vi "2023_day10_Task2.vi"() -> ()   [LabVIEW 2021]
uses:
  458e69ee-25d3-45f1-b600-9235034e037f.vi
  86f884ac-d13f-4936-887d-a05db3f6c1aa.vi
  <vilib>/Array/Sort 2D Array - Pop Stack.vi
  <vilib>/Array/Sort 2D Array - Push Stack.vi
  458e69ee-25d3-45f1-b600-9235034e037f.vi/269d4b3b-47f5-49e3-8884-44851e4dd9d5.vi
  458e69ee-25d3-45f1-b600-9235034e037f.vi/6d99389c-673d-4efb-bf33-19b32bcf4cf8.vi
  86f884ac-d13f-4936-887d-a05db3f6c1aa.vi/269d4b3b-47f5-49e3-8884-44851e4dd9d5.vi
  86f884ac-d13f-4936-887d-a05db3f6c1aa.vi/6d99389c-673d-4efb-bf33-19b32bcf4cf8.vi
panel:
  out "Character Array":string[][](array[string])
  out "Array":i32[](array[numeric])
  out "Numeric 3":i32
  out "sorted 2D array":i32[][](array[numeric])
  out "XY Graph":cluster{"Numeric":i32, "Numeric":i32}[](graph)
  in  "Switch":bool caption="Ex. Data  vs.  User Data"
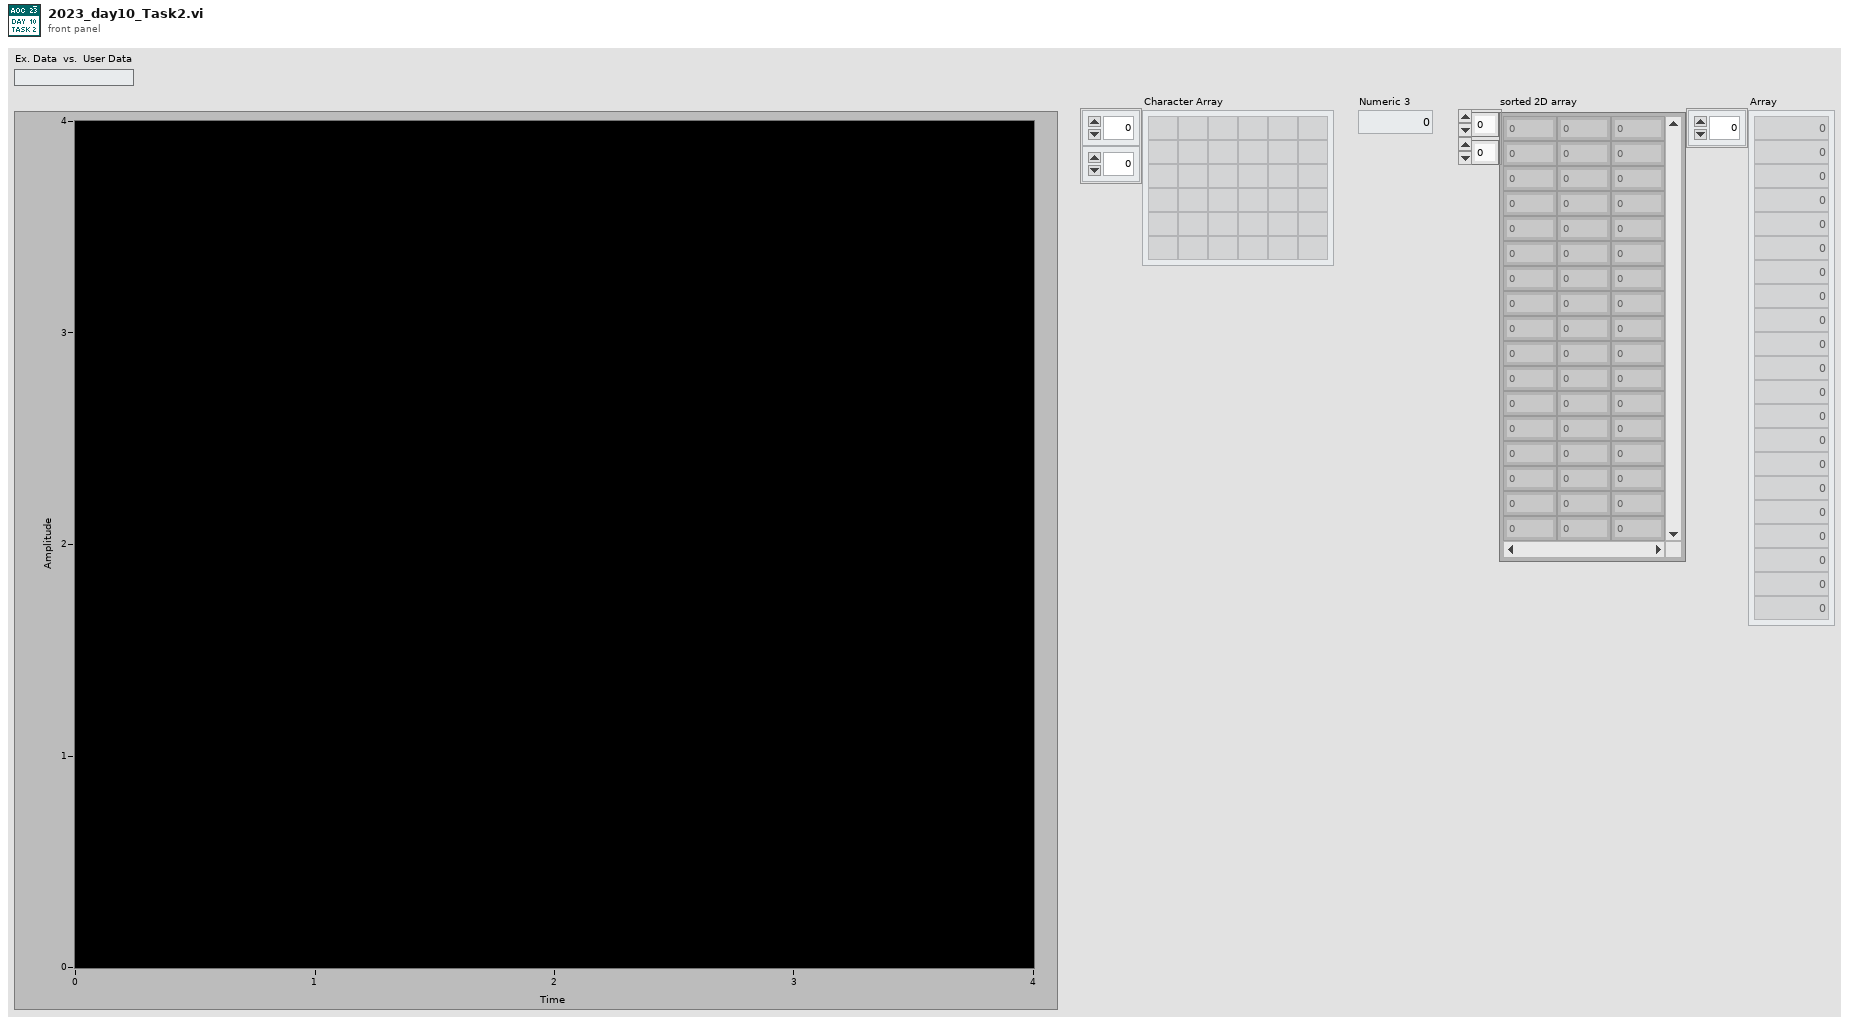
[diagram p1: front panel]
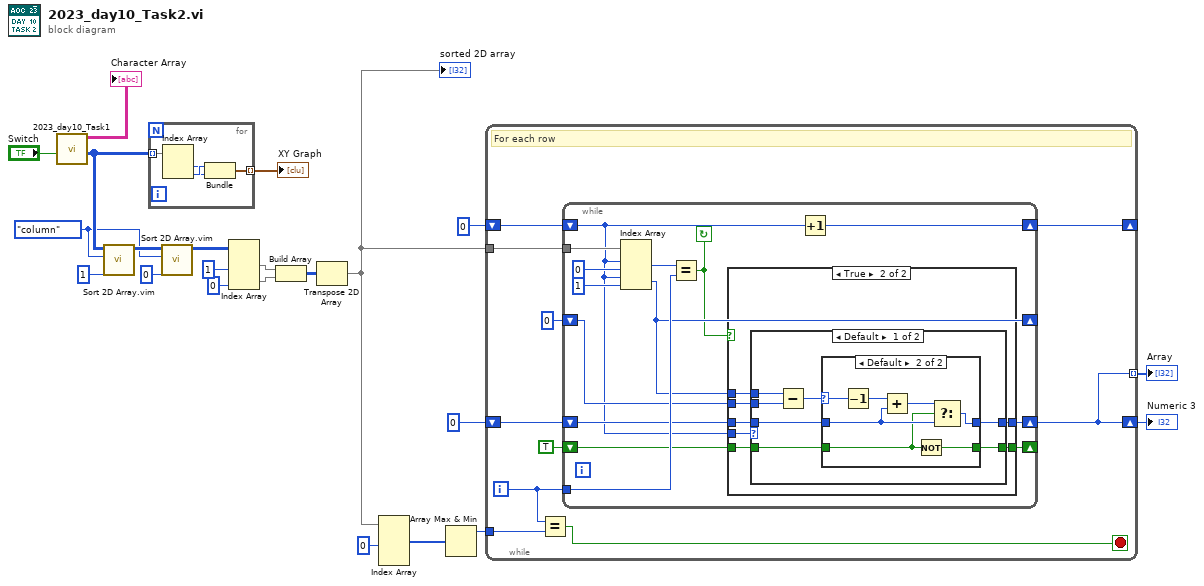
[diagram p0: block diagram]
diagram:
  w9 = enum16{"column", "row"}."column" ("dimension to index (column)")
  n1 = call "2023_day10_Task1.vi"("Switch"="Switch") -> ("Curve Points"=w20:i32[][], "Character Array"=→"Character Array":string[][])  [unwired: 9 in]
  n2 = call "Sort 2D Array.vim"("index"=1, "dimension to index (column)"=w9, "2D array"=w20) -> ("sorted 2D array"=w17:i32[][])  [unwired: 7 in, 1 out]
  n3 = for {
    tunnel: w20 -> [w26] mode=indexing
    tunnel: [w23] -> w21 mode=indexing
    n4 = Index Array(array=w26) -> (element #1=w24:i32, element #2=w25:i32)  [unwired: 2 in]
    n5 = Bundle("Numeric"=w25, "Numeric"=w24) -> (w23:cluster{"Numeric":i32, "Numeric":i32})  [unwired: 1 in]
  }
  "XY Graph" <- w21
  n6 = call "Sort 2D Array.vim"("index"=0, "dimension to index (column)"=w9, "2D array"=w17) -> ("sorted 2D array"=w7:i32[][])  [unwired: 7 in, 1 out]
  n7 = Index Array(array=w7, index (col) #1=1 ("disabled index (col)"), index (col) #2=0 ("index (col)")) -> (element #1=w4:i32[], element #2=w3:i32[])  [unwired: 2 in]
  n8 = Build Array(w4, w3) -> (w2:i32[][])
  n9 = Transpose 2D Array(2D array=w2) -> (transposed array=w1:i32[][])
  "sorted 2D array" <- w1
  n10 = Index Array(array=w1, index (col) #1=0 ("disabled index (col)")) -> (element #1=w12:i32[])  [unwired: 3 in, 1 out]
  n11 = Array Max & Min(array=w12) -> (max value=w11:i32)  [unwired: 3 out]
  n12 = while {
    tunnel: w1 -> [w36]
    shift-right: [w32] -> w15
    shift-left: 0 -> [w33]
    tunnel: [w32] -> w14 mode=indexing
    tunnel: w11 -> [w30]
    shift-right: [w27] -> _
    shift-left: 0 -> [w28]
    i -> [w31]
    stop <- w29 stop-if-true
    # "For each row"
    n13 = Equal?(x=w31, y=w30) -> (x = y?=w29:bool)
    n14 = while {
      tunnel: w36 -> [w50]
      tunnel: w31 -> [w47]
      shift-right: [w40] -> _
      shift-left: 0 ("Numeric") -> [w45]
      shift-right: [w44] -> _
      shift-left: TRUE -> [w43]
      shift-right: [w41] -> w32
      shift-left: w33 -> [w42]
      shift-right: [w37] -> w27
      shift-left: w28 -> [w38]
      stop <- w39 continue-if-true
      n15 = Index Array(array=w50, index (row) #1=w38, index (col) #1=0 ("disabled index (col)"), index (row) #2=w38, index (col) #2=1 ("disabled index (col)")) -> (element #1=w48:i32, element #2=w40:i32)
      n16 = Equal?(x=w48, y=w47) -> (x = y?=w39:bool)
      n17 = case shown="True" w39 {
        tunnel: w38 -> [_ w59]
        tunnel: w45 -> [_ w58]
        tunnel: [w51 w57] -> w44
        tunnel: w43 -> [w51 w56]
        tunnel: w42 -> [w52 w55]
        tunnel: [w52 w54] -> w41
        tunnel: w40 -> [_ w53]
        frame False {
        }
        frame True {
          n18 = case shown="Default" w59 {
            tunnel: w58 -> [w66 _]
            tunnel: w53 -> [w65 _]
            tunnel: [w63 w76] -> w57
            tunnel: w56 -> [w62 w76]
            tunnel: w55 -> [w61 w77]
            tunnel: [w60 w77] -> w54
            frame Default {
              n19 = Subtract(x=w65, y=w66) -> (x-y=w64:i32)
              n20 = case shown="Default" w64 {
                selector: w64 -> [_ w75]
                tunnel: [w68 w69] -> w63
                tunnel: w62 -> [w68 w70]
                tunnel: w61 -> [w67 w74]
                tunnel: [w67 w72] -> w60
                frame 0, 1 {
                }
                frame Default {
                  n21 = Decrement(x=w75) -> (x-1=w71:i32)
                  n22 = Add(x=w71, y=w74) -> (x+y=w73:i32)
                  n23 = Not(x=w70) -> (.not. x?=w69:bool)
                  n24 = Select(t=w73, s=w70, f=w74) -> (s? t:f=w72:i32)
                }
              }
            }
            frame 0 {
            }
          }
        }
      }
      n25 = Increment(x=w38) -> (x+1=w37:i32)
    }
  }
  "Numeric 3" <- w15
  "Array" <- w14
